vi "LaunchProcess.vi"(11 "SMO Reference":refnum<class "SMO.lvclass">) -> ()   [LabVIEW 2021, in "smo.lvlib" / "SMO.lvclass"]
doc: "Launches the Process VIs.\n\n---------------------------------------------------------------\nJKI State Machine Objects™\nhttp://jki.net/state-machine-objects/\nCopyright (C) 2005-2015, JKI <info@jki.net>\nALL RIGHTS RESERVED"
uses:
  SMO.lvclass
  SMO.lvclass/SMO.ctl
  Typedefs/SMOState --Enum.ctl
  ReftoDVR--SMO.vi
panel:
  # "For instructions on how to use the JKI State Machine Objects, examples and video tutorials, visit:\nhttp://jki.net/state-machine-objects/\n\nJKI State Machine Objects™\nhttp://jki.net/state-machine-objects/\nCopyright (C) 2005-2015, JKI <info@jki.net>\nALL RIGHTS RESERVED"
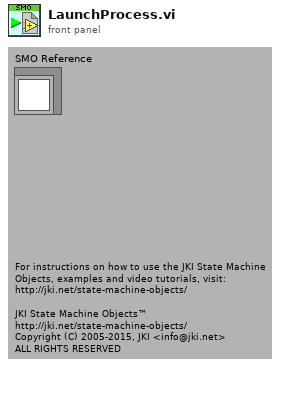
[diagram p1: front panel]
types:
  T1 = typedef "smo.lvlib/SMO.lvclass/SMOState --Enum.ctl" = enum16{"unknown", "Created", "Started", "Stopped"}
  T2 = typedef "SMO.lvclass/SMOState --Enum.ctl" = enum16{"unknown", "Created", "Started", "Stopped"}
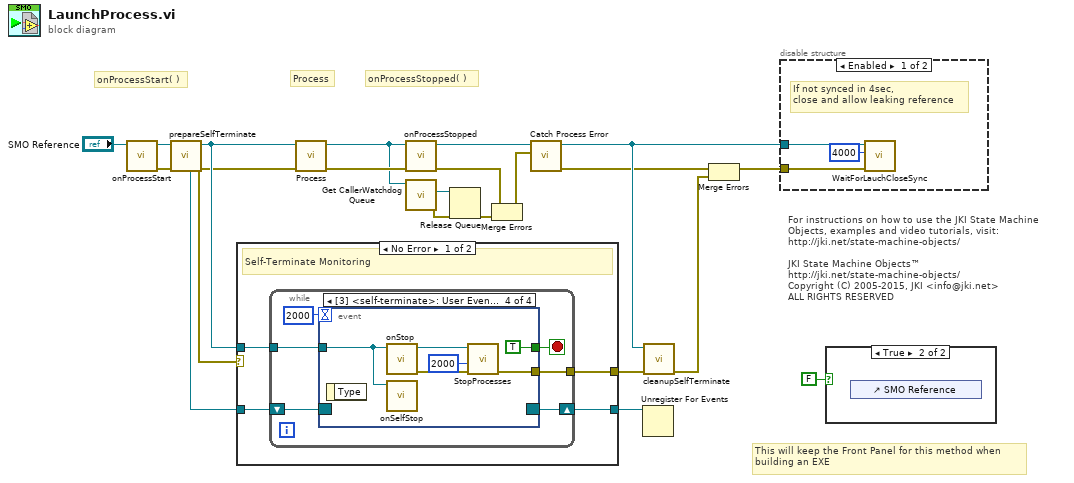
[diagram p0: block diagram]
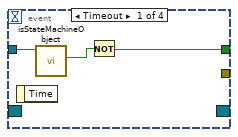
[diagram p2: hidden frame]
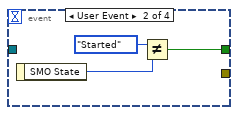
[diagram p3: hidden frame]
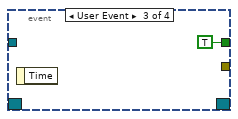
[diagram p4: hidden frame]
diagram:
  # "Process"
  # "onProcessStart( )"
  # "onProcessStopped( )"
  # "This will keep the Front Panel for this method when\nbuilding an EXE"
  # "For instructions on how to use the JKI State Machine Objects, examples and video tutorials, visit:\nhttp://jki.net/state-machine-objects/\n\nJKI State Machine Objects™\nhttp://jki.net/state-machine-objects/\nCopyright (C) 2005-2015, JKI <info@jki.net>\nALL RIGHTS RESERVED"
  n1 = call-dynamic "onProcessStart.vi"("SMO"="SMO Reference") -> ("error out"=w12:errorcluster, "SMO out"=w13:refnum<class "SMO.lvclass">)  [unwired: 9 in]
  n2 = call "prepareSelfTerminate.vi"("error in (no error)"=w12, "SMO in"=w13) -> ("error out"=w9:errorcluster, "SMO out"=w10:refnum<class "SMO.lvclass">, "SelfTerminate EventReg"=w11:refnum<event-registration>)  [unwired: 7 in]
  n3 = case shown="No Error" w9 {
    tunnel: w11 -> [w25 w45]
    tunnel: w10 -> [w24 _]
    tunnel: [w23 w45] -> w5
    tunnel: [w22 _] -> w6
    frame No Error {
      # "Self-Terminate Monitoring"
      n4 = while {
        shift-right: [w30] -> w23
        shift-left: w25 -> [w31]
        tunnel: w24 -> [w27]
        tunnel: [w26] -> w22
        stop <- w28 stop-if-true
        n5 = event shown="[3] <self-terminate>: User Event" {
          selector: w31 -> [_ _ _ _]
          dyn-events: [_ _ _ _] -> w30
          timeout: 2000 -> [_ _ _ _]
          tunnel: [w33 w35 TRUE TRUE] -> w28
          tunnel: w27 -> [w34 _ _ w39]
          tunnel: [_ _ _ w40] -> w26
          event Timeout {
            n6 = event-data() -> ()  [unwired: 1 in, 1 out]
            n7 = call "isStateMachineObject.vi"("SMO"=w34) -> ("is SMO?"=w32:bool)  [unwired: 8 in, 2 out]
            n8 = Not(x=w32) -> (.not. x?=w33:bool)
          }
          event User Event {
            n9 = event-data() -> ("SMO State"=w37:T2)  [unwired: 1 in]
            n10 = Not Equal?(x=SMOState_--Enum."Started", y=w37) -> (x != y?=w35:bool)
          }
          event User Event {
            n11 = event-data() -> ()  [unwired: 1 in, 1 out]
          }
          event User Event {
            n12 = event-data() -> ()  [unwired: 1 in, 1 out]
            n13 = call-dynamic "onStop.vi"("SMO"=w39) -> ("error out"=w42:errorcluster, "SMO out"=w43:refnum<class "SMO.lvclass">)  [unwired: 9 in]
            n14 = call-dynamic "onSelfStop.vi"("SMO"=w39) -> ()  [unwired: 11 in]
            n15 = call "StopProcesses.vi"("error in (no error)"=w42, "timeout in ms (-1)"=2000, "SMO"=w43) -> ("error out"=w40:errorcluster)  [unwired: 7 in, 1 out]
          }
        }
      }
    }
    frame Error {
    }
  }
  n16 = call-dynamic "Process.vi"("error in"=w9, "SMO"=w10) -> ("error out"=w8:errorcluster, "SMO out"=w7:refnum<class "SMO.lvclass">)  [unwired: 8 in]
  n17 = call-dynamic "onProcessStopped.vi"("error in (no error)"=w8, "SMO"=w7) -> ("error out"=w16:errorcluster, "SMO out"=w20:refnum<class "SMO.lvclass">)  [unwired: 8 in]
  n18 = call "Get CallerWatchdog Queue.vi"("SMO in"=w7) -> ("error out"=w18:errorcluster, "Caller Watchdog"=w19:refnum<queue>)  [unwired: 8 in, 1 out]
  n19 = Release Queue(queue=w19, error in (no error)=w18) -> (error out=w17:errorcluster)  [unwired: 1 in, 2 out]
  n20 = Merge Errors(w16, w17) -> (w15:errorcluster)
  n21 = call "Catch Process Error.vi"("Process Error"=w15, "SMO"=w20) -> ("error out"=w2:errorcluster, "SMO out"=w4:refnum<class "SMO.lvclass">)  [unwired: 8 in]
  n22 = Unregister For Events(event registration refnum=w5) -> ()  [unwired: 1 in, 1 out]
  n23 = call "cleanupSelfTerminate.vi"("error in (no error)"=w6, "SMO in"=w4) -> ("error out"=w3:errorcluster)  [unwired: 9 in]
  n24 = Merge Errors(w2, w3) -> (w1:errorcluster)
  n25 = disable-structure shown="Enabled" {
    disable-tunnel: w4 -> [w48 _]
    disable-tunnel: w1 -> [w46 _]
    frame Enabled {
      # "If not synced in 4sec, \nclose and allow leaking reference"
      n26 = call "WaitForLauchCloseSync.vi"("error in (no error)"=w46, "timeout in ms (-1)"=4000, "SMO"=w48) -> ()  [unwired: 7 in, 2 out]
    }
    frame Disabled {
    }
  }
  n27 = case shown="True" FALSE {
    frame False {
    }
    frame True {
      n28 = control-ref of="SMO Reference"() -> ()  [unwired: 1 out]
    }
  }
